vi "Write TraceMessage.vi"(8 "error in (no error)":errorcluster, 10 "TraceMessage.lvclass":refnum<class "Trace.lvclass">, 11 "Tracer in":refnum<class "Tracer.lvclass">) -> (0 "error out":errorcluster, 3 "Tracer out":refnum<class "Tracer.lvclass">)   [LabVIEW 2013, in "Tracer.lvclass"]
uses:
  Tracer.lvclass
  TraceMessage/Trace.lvclass
  Tracer.lvclass/Tracer.ctl
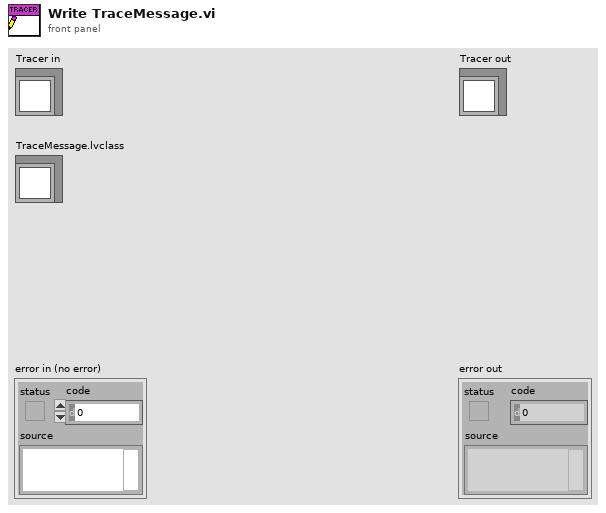
[diagram p1: front panel]
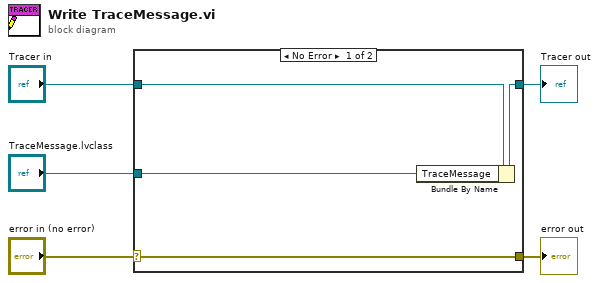
[diagram p0: block diagram]
diagram:
  n1 = case shown="No Error" "error in (no error)" {
    selector: "error in (no error)" -> [w9 w10]
    tunnel: [w9 w10] -> w4
    tunnel: [w7 w11] -> w2
    tunnel: "Tracer in" -> [w8 w11]
    tunnel: "TraceMessage.lvclass" -> [w6 _]
    frame No Error {
      n2 = Bundle By Name(cluster=w8, "TraceMessage"=w6) -> (w7:refnum<class "Tracer.lvclass">)
    }
    frame Error {
    }
  }
  "error out" <- w4
  "Tracer out" <- w2
